vi "Main.vi"(8 "Error In":errorcluster, 11 "New Error (To Be Displayed To User)":T1) -> (0 "Error Out":errorcluster)   [LabVIEW 2023, in "Error Manager.lvlib" / "New Error Dialogue GUI.lvlib"]
doc: "This is a modal, dialogue GUI that displays to the user the error code and error message of a \"new error\" that occured in their application.\n\nPlease note: not necessarily every error that occurs in an application will be displayed by this dialogue. For example, if a while loop in an application starts producing an error in a loop, and starts spamming the Error Manager module with dozens or hundreds of errors every second, we don't want this GUI to pop-up once for every such error. That's why this GUI displays only \"New Errors\".\n\nTo find the definition of a \"New Error\", find the place in the main Error Manager module that enqueues the command that triggers this GUI to pop-up. The logic that determines whether a message should be enqueued or not is the logic that defines a \"New Error\"."
uses:
  New Error Dialogue GUI.lvlib
  Module Data - Outputs (cluster).ctl
  New Error (To Be Displayed To User) (cluster).ctl
  MHL Queue/Command (enum).ctl
  <vilib>/Utility/error.llb/DialogType.ctl
  Stop EHL (library variable).vi
  Module Data (cluster).ctl
  MHL Queue/MHL Queue.lvlib
  Module Data - Work (cluster).ctl
  Module Data - Inputs (cluster).ctl
  Error Manager.lvlib
panel:
  out "Error Message":string
  out "Error Code":i32
  in  "Sizing Tool":bool
  out "Outputs":T2
  in  "OK":bool
  out "MHL iteration":i32
  out "EHL iteration":i32
  out "Error Out":errorcluster
  # "#TemplateNote\nThe front panel region that will be displayed to the user is determined by the pale green and pale red square boxes. These square boxes act as markers that allow a subVI to resize the front panel to the desired dimensions.\n\nThe pale green square box represents the top-left of the user-visible region, while the pale red box represents the bottom-right corner of what the user can see.\n\nWhen developing, move the boxes to adjust the user-visible region as desired. The markers make the resizing a much quicker, visual and more intuitive process."
  # "#TemplateNote\nThis is the Modal Dialogue Template\n\nFor details, see the block diagram comments."
  # "User-visible Region"
  # "Error"
  # "Region invisible to the user"
  # "Input\nInputs to the VI"
  # "Development\ncontrols/indicators useful for development and testing, but which are not outputs of the VI"
  # "Output\nOutputs of the VI"
  # "The Error Out indicator is larger than usual in order to be able to view the full error message without having to scroll."
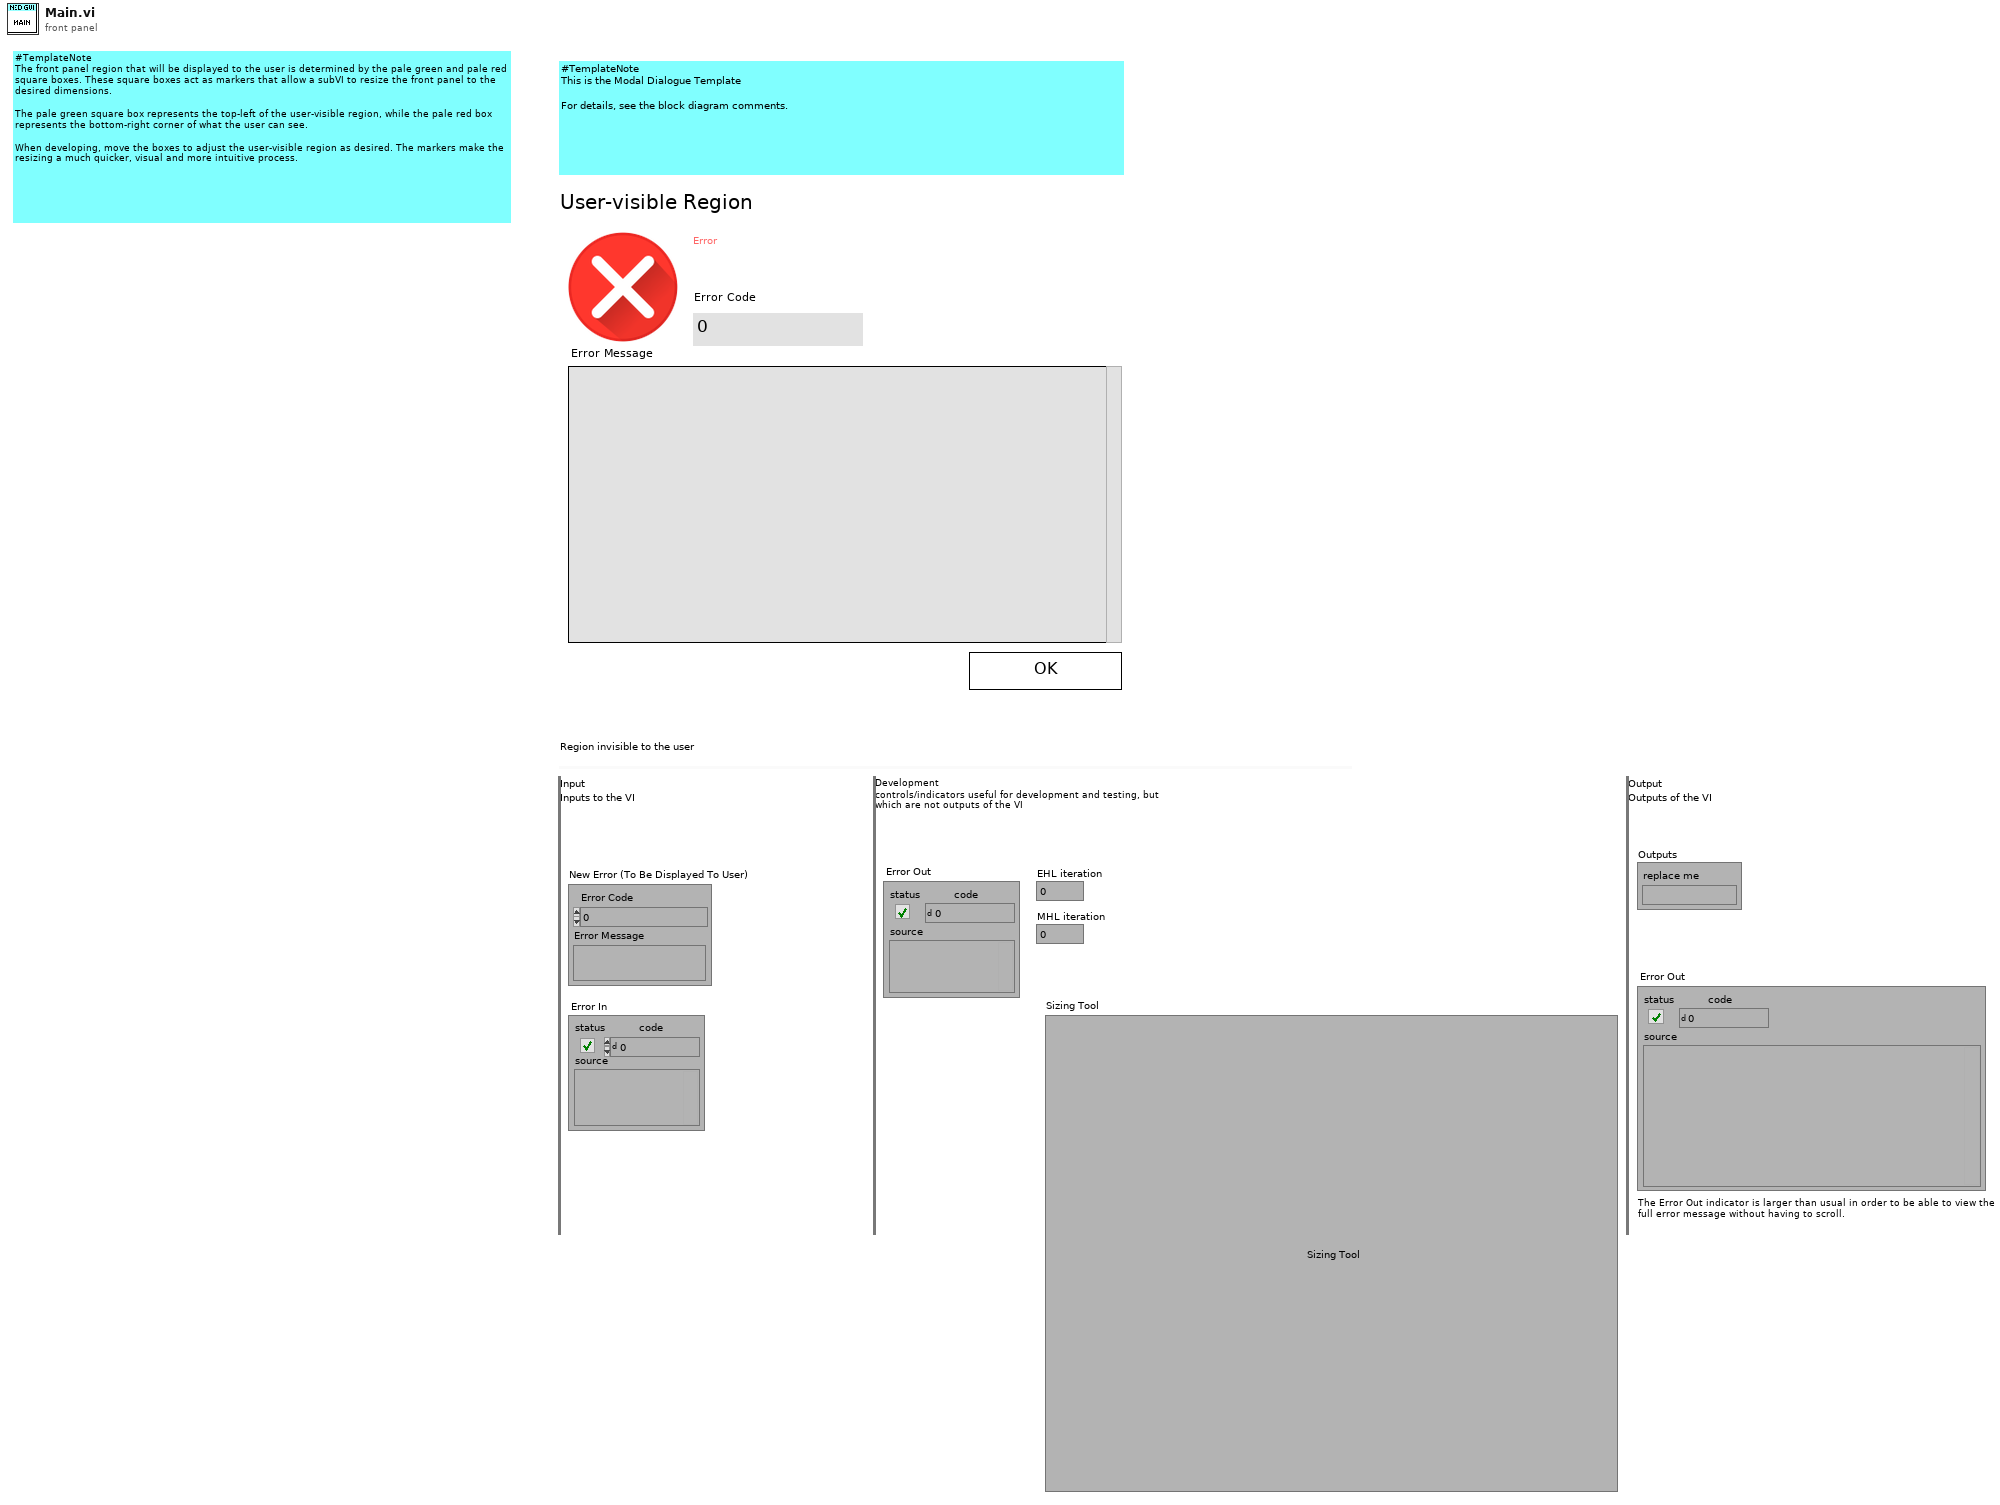
[diagram p1: front panel]
types:
  T1 = typedef "Error Manager.lvlib/New Error Dialogue GUI.lvlib/New Error (To Be Displayed To User) (cluster).ctl" = cluster{"Error Code":i32, "Error Message":string}
  T2 = typedef "Error Manager.lvlib/New Error Dialogue GUI.lvlib/Module Data - Outputs (cluster).ctl" = cluster{"replace me":string}
  T3 = typedef "Error Manager.lvlib/New Error Dialogue GUI.lvlib/MHL Queue.lvlib/Command (enum).ctl" = enum16{"Init Module", "Close Module", "Handle Local Error", "OK Button Pressed"}
  T4 = typedef "Error Manager.lvlib/New Error Dialogue GUI.lvlib/Module Data - Work (cluster).ctl" = cluster{"replace me":string}
  T5 = typedef "Error Manager.lvlib/New Error Dialogue GUI.lvlib/Module Data - Inputs (cluster).ctl" = cluster{"replace me":string}
  T6 = typedef "Error Manager.lvlib/New Error Dialogue GUI.lvlib/Module Data (cluster).ctl" = cluster{"Inputs":T5, "Work":T4, "Outputs":T2}
  T7 = typedef "DialogType.ctl" = u16
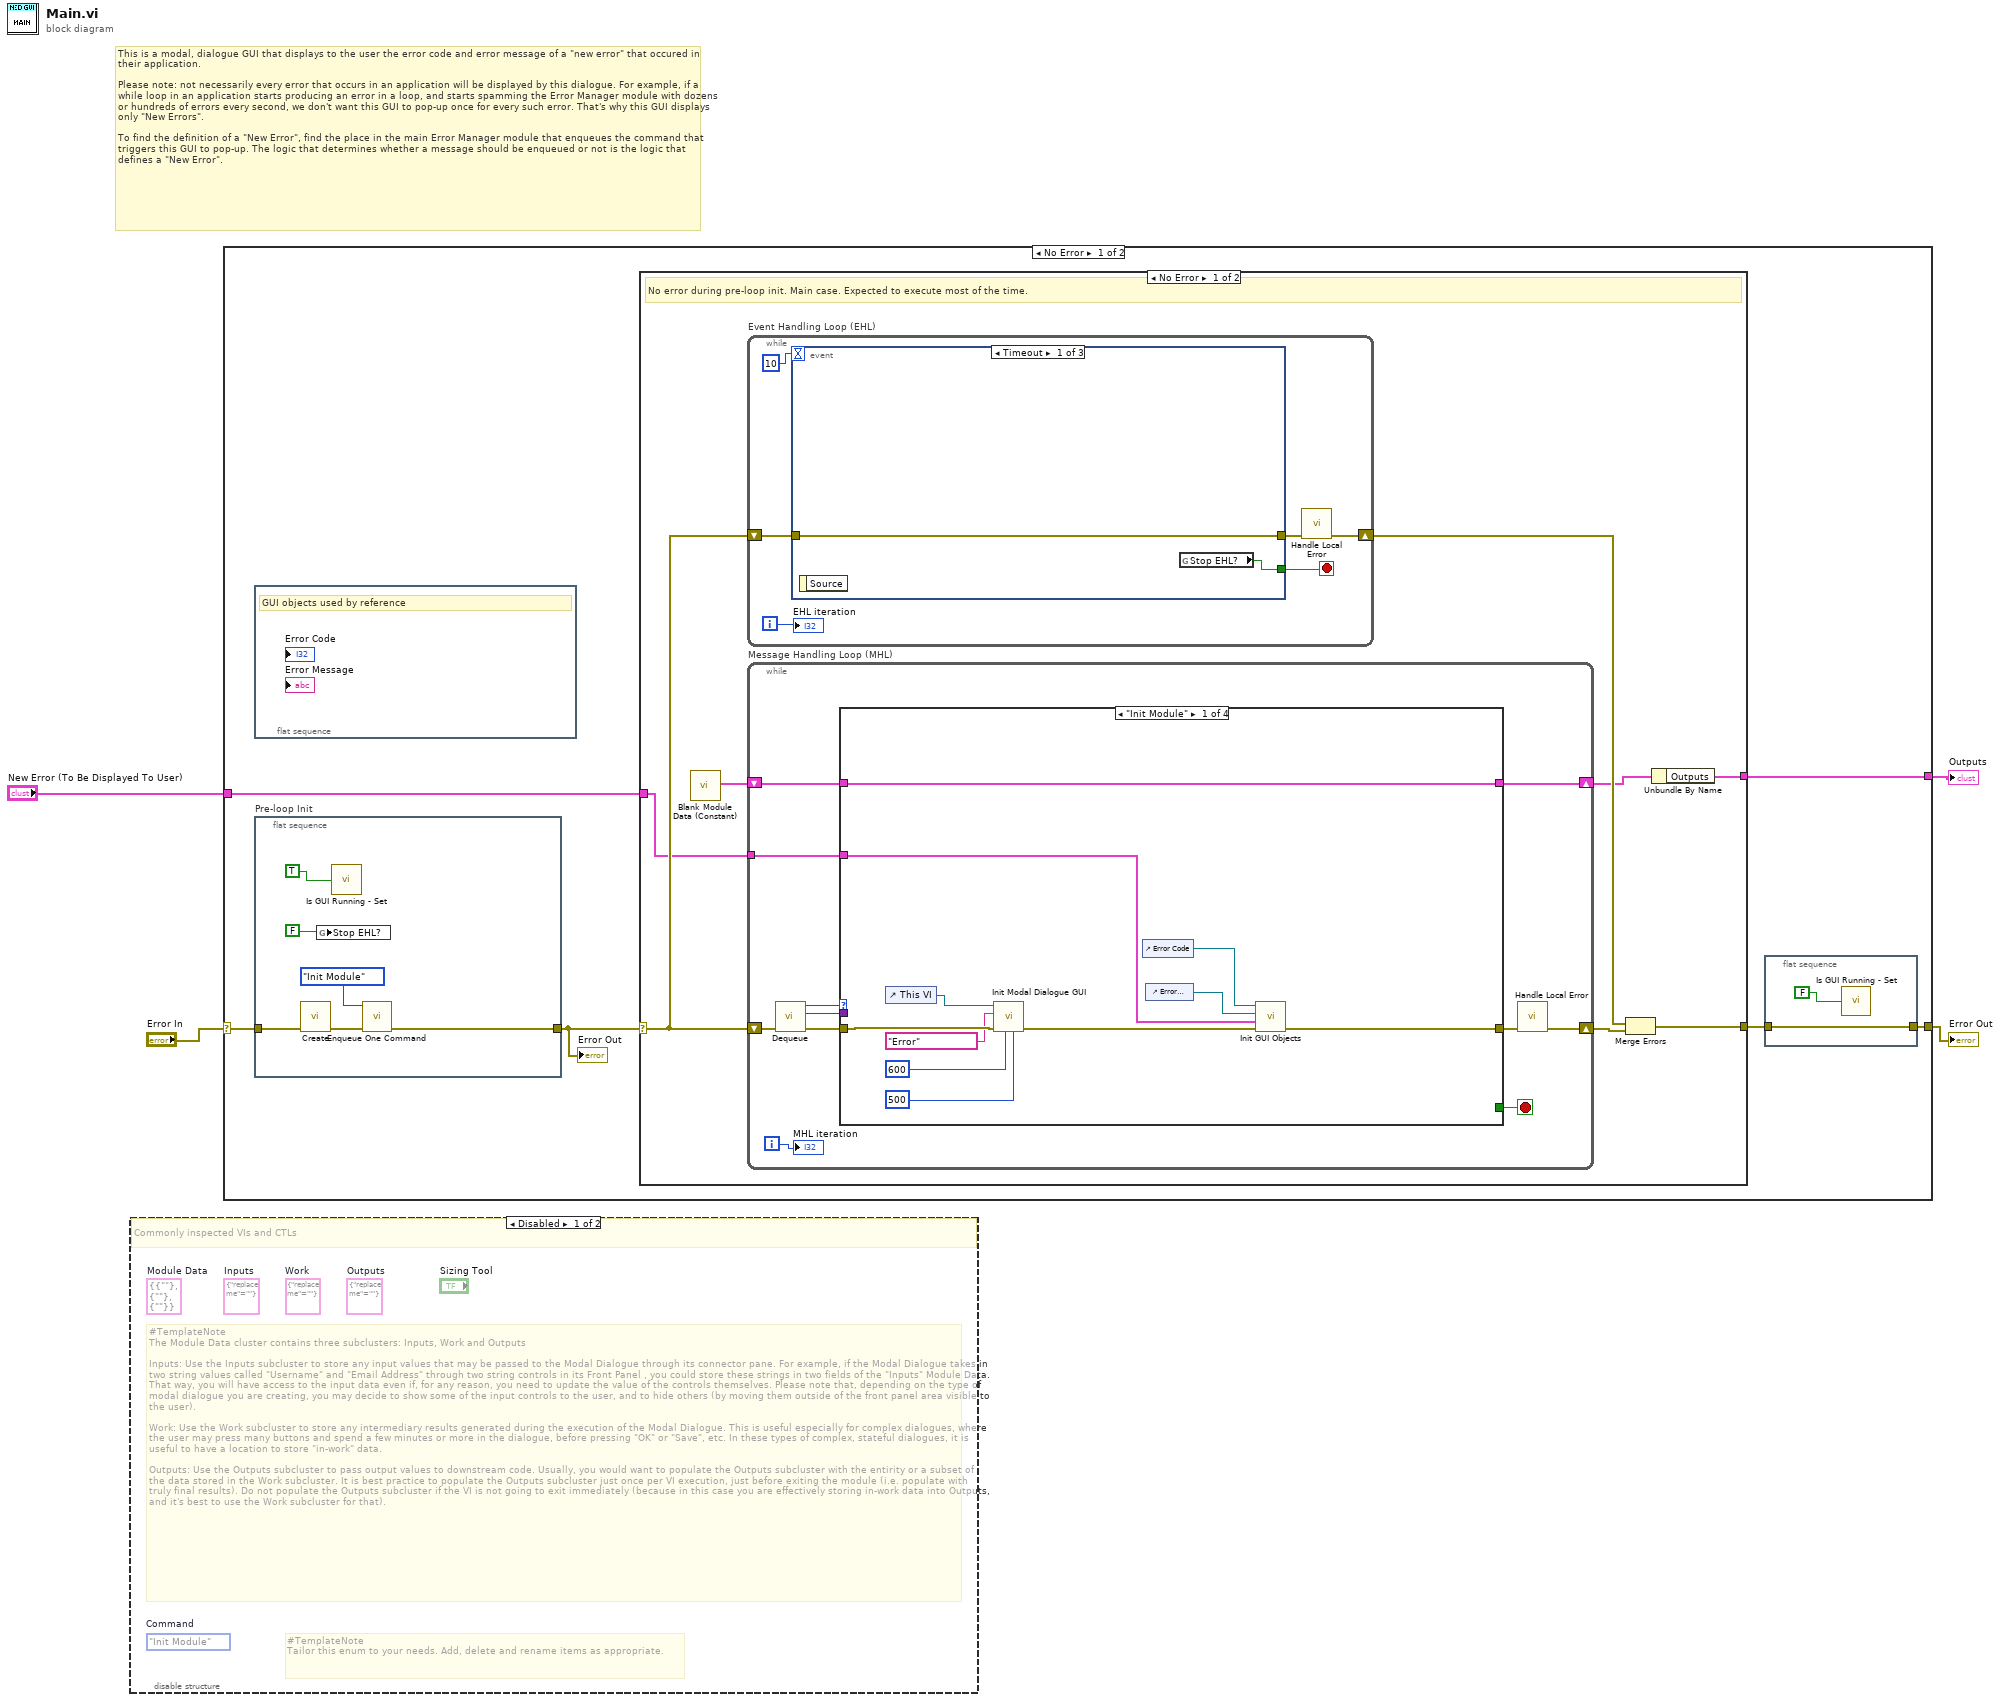
[diagram p0: block diagram]
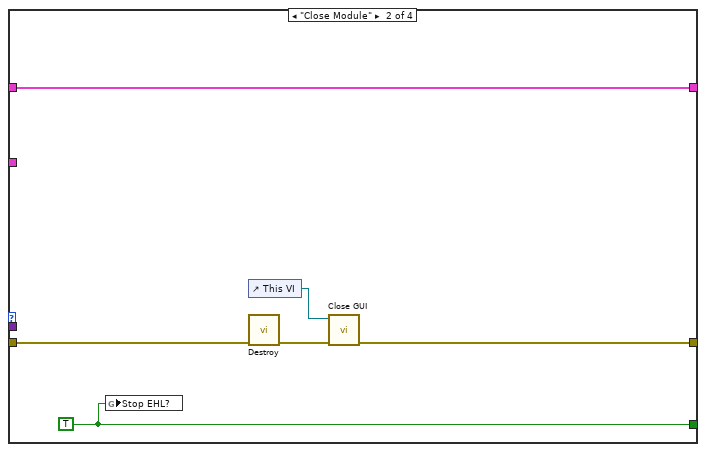
[diagram p2: hidden frame]
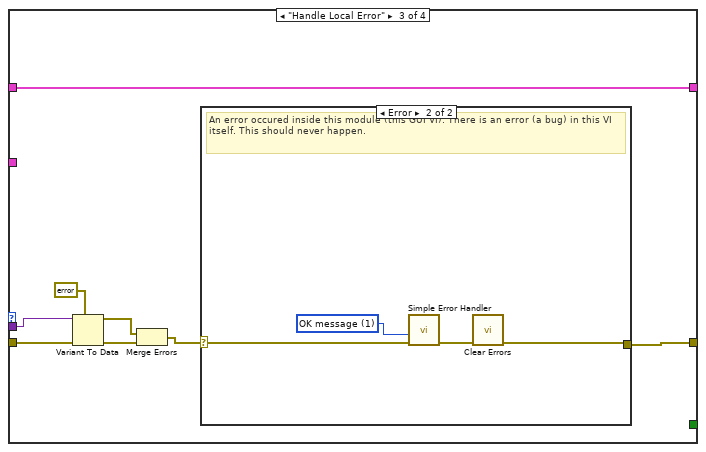
[diagram p3: hidden frame]
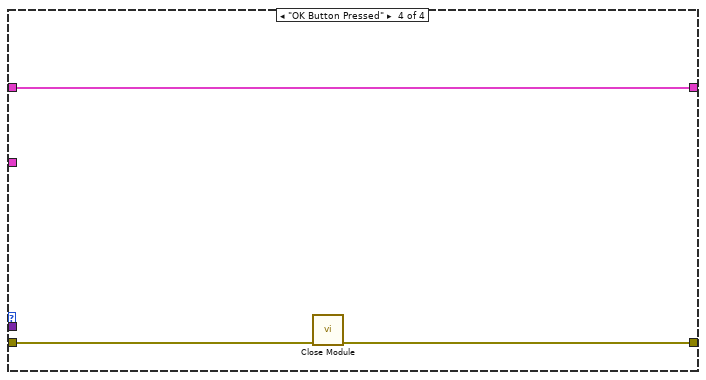
[diagram p5: hidden frame]
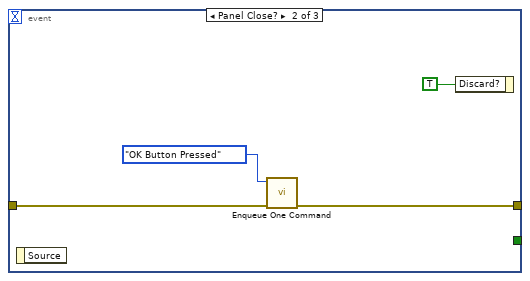
[diagram p6: hidden frame]
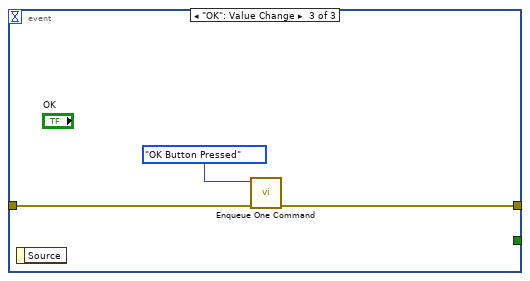
[diagram p7: hidden frame]
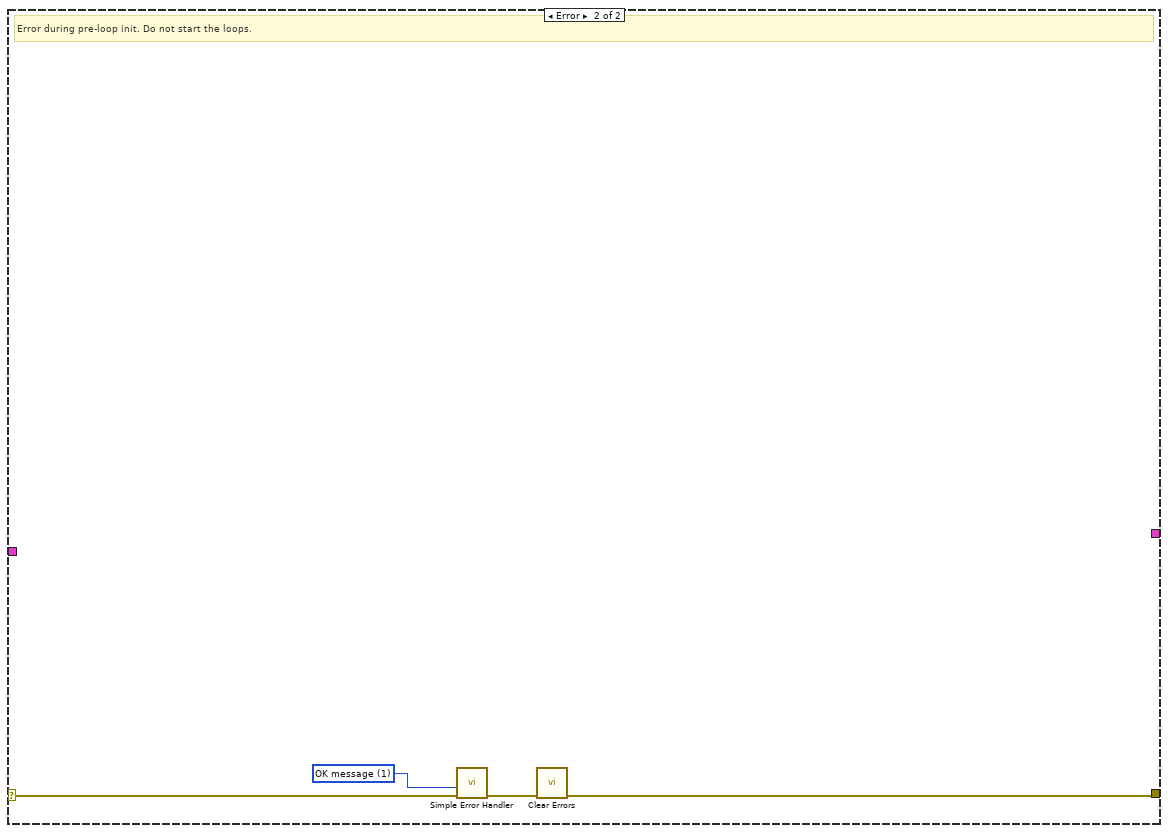
[diagram p8: hidden frame]
diagram:
  # "This is a modal, dialogue GUI that displays to the user the error code and error message of a \"new error\" that occured in their application.\n\nPlease note: not necessarily every error that occurs in an application will be displayed by this dialogue. For example, if a while loop in an application starts producing an error in a loop, and starts spamming the Error Manager module with dozens or hundreds of errors every second, we don't want this GUI to pop-up once for every such error. That's why this GUI displays only \"New Errors\".\n\nTo find the definition of a \"New Error\", find the place in the main Error Manager module that enqueues the command that triggers this GUI to pop-up. The logic that determines whether a message should be enqueued or not is the logic that defines a \"New Error\"."
  n1 = disable-structure shown="Disabled" {
    frame Disabled {
      (unwired) Command_(enum)."Init Module"  # Command
      (unwired) T2 {"replace me"=""}  # Outputs
      (unwired) T4 {"replace me"=""}  # Work
      (unwired) T5 {"replace me"=""}  # Inputs
      (unwired) T6 {"Inputs"={"replace me"=""}, "Work"={"replace me"=""}, "Outputs"={"replace me"=""}}  # Module Data
      # "#TemplateNote\nTailor this enum to your needs. Add, delete and rename items as appropriate."
      # "#TemplateNote\nThe Module Data cluster contains three subclusters: Inputs, Work and Outputs\n\nInputs: Use the Inputs subcluster to store any input values that may be passed to the Modal Dialogue through its connector pane. For example, if the Modal Dialogue takes in two string values called \"Username\" and \"Email Address\" through two string controls in its Front Panel , you could store these strings in two fields of the \"Inputs\" Module Data. That way, you will have access to the input data even if, for any reason, you need to update the value of the controls themselves. Please note that, depending on the type of modal dialogue you are creating, you may decide to show some of the input controls to the user, and to hide others (by moving them outside of the front panel area visible to the user).\n\nWork: Use the Work subcluster to store any intermediary results generated during the execution of the Modal Dialogue. This is useful especially for complex dialogues, where the user may press many buttons and spend a few minutes or more in the dialogue, before pressing \"OK\" or \"Save\", etc. In these types of complex, stateful dialogues, it is useful to have a location to store \"in-work\" data.\n\nOutputs: Use the Outputs subcluster to pass output values to downstream code. Usually, you would want to populate the Outputs subcluster with the entirity or a subset of the data stored in the Work subcluster. It is best practice to populate the Outputs subcluster just once per VI execution, just before exiting the module (i.e. populate with truly final results). Do not populate the Outputs subcluster if the VI is not going to exit immediately (because in this case you are effectively storing in-work data into Outputs, and it's best to use the Work subcluster for that)."
      # "Commonly inspected VIs and CTLs"
    }
    frame Enabled {
    }
  }
  n2 = case shown="No Error" "Error In" {
    selector: "Error In" -> [w9 w90]
    tunnel: [w5 w90] -> w4
    tunnel: [w8 _] -> w2
    tunnel: "New Error (To Be Displayed To User)" -> [w7 _]
    frame No Error {
      n3 = flat-sequence {
        frame #0 {
          # "GUI objects used by reference"
        }
      }
      n4 = flat-sequence "Pre-loop Init" {
        tunnel: [w17] -> w10
        tunnel: w9 -> [w14]
        frame #0 {
          n5 = call "Create.vi"("error in (no error)"=w14) -> ("error out"=w18:errorcluster)  [unwired: 10 in]
          n6 = global write "Stop EHL (library variable).vi" "Stop EHL?"(FALSE) -> ()
          n7 = call "Is GUI Running - Set.vi"("Is GUI Running?"=TRUE) -> ()
          n8 = call "Enqueue One Command.vi"("error in (no error)"=w18, "Command"=Command_(enum)."Init Module") -> ("error out"=w17:errorcluster)  [unwired: 9 in]
        }
      }
      n9 = case shown="No Error" w10 {
        selector: w10 -> [w24 w89]
        tunnel: [w19 w87] -> w6
        tunnel: [w22 _] -> w8
        tunnel: w7 -> [w20 _]
        frame No Error {
          # "No error during pre-loop init. Main case. Expected to execute most of the time."
          n10 = call "Blank Module Data (Constant).vi"() -> ("Blank Module Data"=w21:T6)
          n11 = while "Event Handling Loop (EHL)" {
            shift-right: [w74] -> w26
            shift-left: w24 -> [w76]
            i -> [w72]
            stop <- w75 stop-if-true
            n12 = event shown="[0] Timeout" {
              selector: _ -> [_ _ _]
              dyn-events: _ -> [_ _ _]
              timeout: 10 -> [_ _ _]
              tunnel: w76 -> [w78 w80 w84]
              tunnel: [w77 _ _] -> w75
              tunnel: [w78 w79 w83] -> w73
              event Timeout {
                n13 = event-data() -> ()  [unwired: 1 in, 1 out]
                n14 = global read "Stop EHL (library variable).vi" "Stop EHL?"() -> (w77:bool)
              }
              event Panel Close? {
                n15 = event-data() -> ()  [unwired: 1 in, 1 out]
                n16 = call "Enqueue One Command.vi"("error in (no error)"=w80, "Command"=Command_(enum)."OK Button Pressed") -> ("error out"=w79:errorcluster)  [unwired: 9 in]
                n17 = event-data("Discard?"=TRUE) -> ()  [unwired: 1 in, 1 out]
              }
              event "OK": Value Change {
                n18 = event-data() -> ()  [unwired: 1 in, 1 out]
                n19 = call "Enqueue One Command.vi"("error in (no error)"=w84, "Command"=Command_(enum)."OK Button Pressed") -> ("error out"=w83:errorcluster)  [unwired: 9 in]
              }
            }
            n20 = call "Handle Local Error.vi"("Error In"=w73) -> ("Error Out"=w74:errorcluster)  [unwired: 10 in]
            "EHL iteration" <- w72
          }
          n21 = while "Message Handling Loop (MHL)" {
            shift-right: [w28] -> w23
            shift-left: w21 -> [w30]
            shift-right: [w34] -> w25
            shift-left: w24 -> [w33]
            tunnel: w20 -> [w27]
            i -> [w31]
            stop <- w37 stop-if-true
            n22 = call "Dequeue.vi"("error in (no error)"=w33) -> ("error out"=w35:errorcluster, "Data"=w32:variant, "Command"=w29:T3)  [unwired: 8 in]
            n23 = case shown="\"Init Module\"" w29 {
              tunnel: w35 -> [w42 w54 w58 w69]
              tunnel: [w47 w50 w57 w68] -> w36
              tunnel: [_ w52 _ _] -> w37
              tunnel: w32 -> [_ _ w56 _]
              tunnel: [w48 w53 w62 w70] -> w28
              tunnel: w30 -> [w48 w53 w62 w70]
              tunnel: w27 -> [w44 _ _ _]
              frame "Init Module" {
                n24 = control-ref of="This VI"() -> (w41:refnum<vi>)
                n25 = call "Init Modal Dialogue GUI.vi"("GUI Vertical Size (pixels)"=i16 500, "GUI Horizontal Size (pixels)"=i16 600, "error in"=w42, "Window Title"="Error", "VI Refnum"=w41) -> ("error out"=w43:errorcluster)  [unwired: 6 in]
                n26 = control-ref of="Error Code"() -> (w46:refnum<vi>)
                n27 = control-ref of="Error Message"() -> (w45:refnum<vi>)
                n28 = call "Init GUI Objects.vi"("error in"=w43, "New Error"=w44, "Error Message"=w45, "Error Code"=w46) -> ("error out"=w47:errorcluster)  [unwired: 7 in]
              }
              frame "Close Module" {
                w52 = TRUE
                n29 = global write "Stop EHL (library variable).vi" "Stop EHL?"(w52) -> ()
                n30 = control-ref of="This VI"() -> (w49:refnum<vi>)
                n31 = call "Destroy.vi"("error in (no error)"=w54) -> ("error out"=w51:errorcluster)  [unwired: 8 in, 2 out]
                n32 = call "Close GUI.vi"("error in"=w51, "VI Refnum"=w49) -> ("error out"=w50:errorcluster)  [unwired: 9 in]
              }
              frame "Handle Local Error" {
                n33 = Variant To Data(error in=w58, type=errorcluster {"status"=FALSE, "code"=0, "source"=""} ("error constant"), Variant=w56) -> (data=w55:errorcluster, error out=w60:errorcluster)
                n34 = Merge Errors(w55, w60) -> (w59:errorcluster)
                n35 = case shown="Error" w59 {
                  selector: w59 -> [w63 w66]
                  tunnel: [w63 w67] -> w57
                  frame No Error {
                  }
                  frame Error {
                    w64 = T7 1 items=["no dialog", "OK message", "continue or stop message", "OK message + warnings", "continue/stop + warnings"] ("type of dialog (OK msg:1)")
                    # "An error occured inside this module (this GUI VI). There is an error (a bug) in this VI itself. This should never happen."
                    n36 = call <vilib>:"Simple Error Handler.vi"("type of dialog (OK msg:1)"=w64, "error in (no error)"=w66) -> ("error out"=w65:errorcluster)  [unwired: 3 in, 4 out]
                    n37 = call <vilib>:"Clear Errors.vi"("error in (no error)"=w65) -> ("error out"=w67:errorcluster)  [unwired: 5 in, 1 out]
                  }
                }
              }
              frame "OK Button Pressed" {
                n38 = call "Close Module.vi"("Error In"=w69) -> ("Error Out"=w68:errorcluster)  [unwired: 10 in]
              }
            }
            n39 = call "Handle Local Error.vi"("Error In"=w36) -> ("Error Out"=w34:errorcluster)  [unwired: 10 in]
            "MHL iteration" <- w31
          }
          n40 = Merge Errors(w26, w25) -> (w19:errorcluster)
          n41 = Unbundle By Name(w23) -> ("Outputs"=w22:T2)
        }
        frame Error {
          w86 = T7 1 items=["no dialog", "OK message", "continue or stop message", "OK message + warnings", "continue/stop + warnings"] ("type of dialog (OK msg:1)")
          # "Error during pre-loop init. Do not start the loops."
          n42 = call <vilib>:"Simple Error Handler.vi"("type of dialog (OK msg:1)"=w86, "error in (no error)"=w89) -> ("error out"=w88:errorcluster)  [unwired: 3 in, 4 out]
          n43 = call <vilib>:"Clear Errors.vi"("error in (no error)"=w88) -> ("error out"=w87:errorcluster)  [unwired: 5 in, 1 out]
        }
      }
      n44 = flat-sequence {
        tunnel: [w12] -> w5
        tunnel: w6 -> [w12]
        frame #0 {
          n45 = call "Is GUI Running - Set.vi"("Is GUI Running?"=FALSE) -> ()
        }
      }
      "Error Out" <- w10
    }
    frame Error {
      # "Error upstream. Do nothing."
    }
  }
  "Error Out" <- w4
  "Outputs" <- w2
